vi "LED Initialization.vi"(8 "Device ID":dbl=-1.0, 11 "CANifier Name":string="UseGlobal") -> ()   [LabVIEW 2019]
uses:
  Globals/LED_Globals.vi
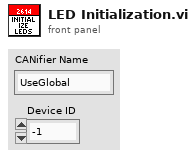
[diagram p1: front panel]
types:
  T1 = enum16{"Off", "NoOp1", "Turret Locked", "NoOp3", "Intaking", "NoOp5", "NoOp6", "Signal Human Player", "NoOp8", "NoOp9", "Firing", "NoOp11", "NoOp12", "NoOp13", "NoOp14", "Climbing - Rainbow"}
  T2 = typedef "CTRE_CANifier_DeviceRef.ctl" = cluster{"DeviceStatus":errorcluster, "Device Number":u8, "Handle":u64, "UsageFrame":u32, "Library Path":path}
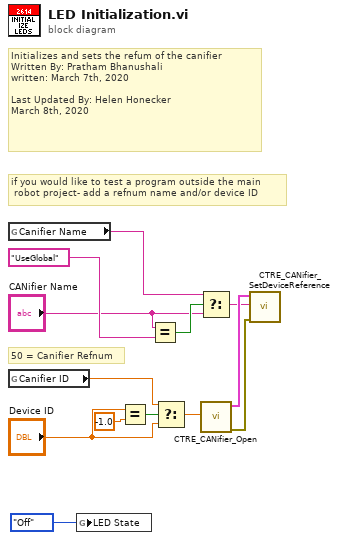
[diagram p0: block diagram]
diagram:
  # "if you would like to test a program outside the main\n robot project- add a refnum name and/or device ID"
  # "50 = Canifier Refnum"
  # "Initializes and sets the refum of the canifier\nWritten By: Pratham Bhanushali\nwritten: March 7th, 2020\n\nLast Updated By: Helen Honecker\nMarch 8th, 2020"
  n1 = global read "LED_Globals.vi" "Canifier Name"() -> (w7:string)
  n2 = global read "LED_Globals.vi" "Canifier ID"() -> (w4:dbl)
  n3 = global write "LED_Globals.vi" "LED State"(T1."Off" ("LED State")) -> ()
  n4 = Equal?(x="Device ID", y=-1.0) -> (x = y?=w10:bool)
  n5 = Equal?(x="CANifier Name", y="UseGlobal") -> (x = y?=w2:bool)
  n6 = Select(t=w4, s=w10, f="Device ID") -> (s? t:f=w8:dbl)
  n7 = Select(t=w7, s=w2, f="CANifier Name") -> (s? t:f=w6:string)
  n8 = call <vilib>:"CTRE_CANifier_Open.vi"("Device Number"=w8) -> ("error out"=w13:errorcluster, "CANifierDevRef"=w12:T2)  [unwired: 9 in]
  n9 = call <vilib>:"CTRE_CANifier_SetDeviceReference.vi"("error in (no error)"=w13, "refnum name"=w6, "CANifierDevRef"=w12) -> ()  [unwired: 7 in, 2 out]
